vi "Trigger Channel.vi"(8 "error in (no error)":errorcluster, 11 "Node Ptr":T1 format="%.0x") -> (0 "error out":errorcluster)   [LabVIEW 2019, in "Instrument Addon System Explorer.lvlib"]
uses:
  Instrument Addon System Explorer.lvlib
  <vilib>/NI VeriStand/Custom Device API/Custom Device Item Ref.ctl
  NationalInstruments.VeriStand.SystemStorageUI
  Addon Shared/Types/FG Control.ctl
  NationalInstruments.VeriStand.SystemStorage
  Addon Shared/SubVIs/Constants.vi
  <vilib>/NI VeriStand/Custom Device API/NI VeriStand - Get Item Property.vi
  <vilib>/NI VeriStand/Custom Device API/Get Item Property (Boolean).vi
  <vilib>/NI VeriStand/Custom Device API/Get Item Property (String).vi
  <vilib>/NI VeriStand/Custom Device API/NI VeriStand - Set Item Property.vi
  <vilib>/NI VeriStand/Custom Device API/Set Item Property (Boolean).vi
  <vilib>/NI VeriStand/Custom Device API/Set Item Property (String).vi
  <vilib>/NI VeriStand/Custom Device API/Custom Device API.lvlib
  <vilib>/NI VeriStand/UI Controls/Single Node Browser/NI_VS UI Single Node Browser.lvlib
  Addon Shared/Instrument Addon Shared.lvlib
panel:
  in  "Header 2":cluster{"Section Name":string}={"Section Name"="Trigger Item Settings"}
  in  "Channel":refnum<k24>(container) caption="Value"
  in  "Use Channel?":bool
  in  "SHDocVw.IWebBrowser":refnum<k7>(container)
  in  "Header":cluster{"Section Name":string}={"Section Name"="Custom Device Item Settings"}
  in  "Description":string
  out "Name":string
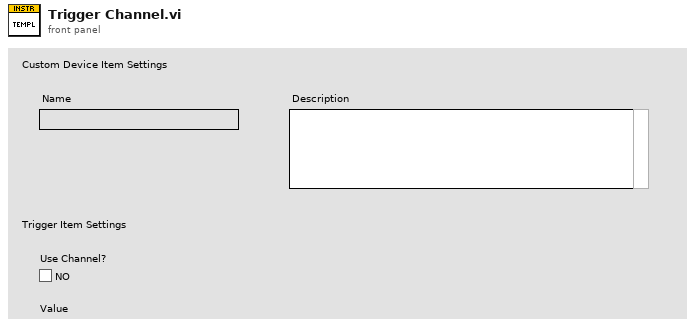
[diagram p1: front panel]
types:
  T1 = typedef "Custom Device API.lvlib/Custom Device Item Ref.ctl" = u64
  T2 = typedef "Instrument Addon Shared.lvlib/FG Control.ctl" = enum16{"Get", "Set"}
  T3 = typedef "Instrument Addon Shared.lvlib/Trigger Parameters.ctl" = cluster{"Use Channel":bool, "Channel Path":string}
  T4 = typedef "Custom Device API.lvlib/Custom Device Item Info.ctl" = cluster{"Name":string, "Is Channel":bool, "GUID":string, "Is Waveform":bool}
  T5 = typedef "Custom Device API.lvlib/Custom Device Commands.ctl" = enum16{"Default", "Item renamed", "Shutdown", "Dynamic button pressed"}
  T6 = typedef "NI_VS UI Single Node Browser.lvlib/Node Ref.ctl" = refnum<k24>
  T7 = typedef "Custom Device API.lvlib/Custom Device Pointer.ctl" = refnum<k24>
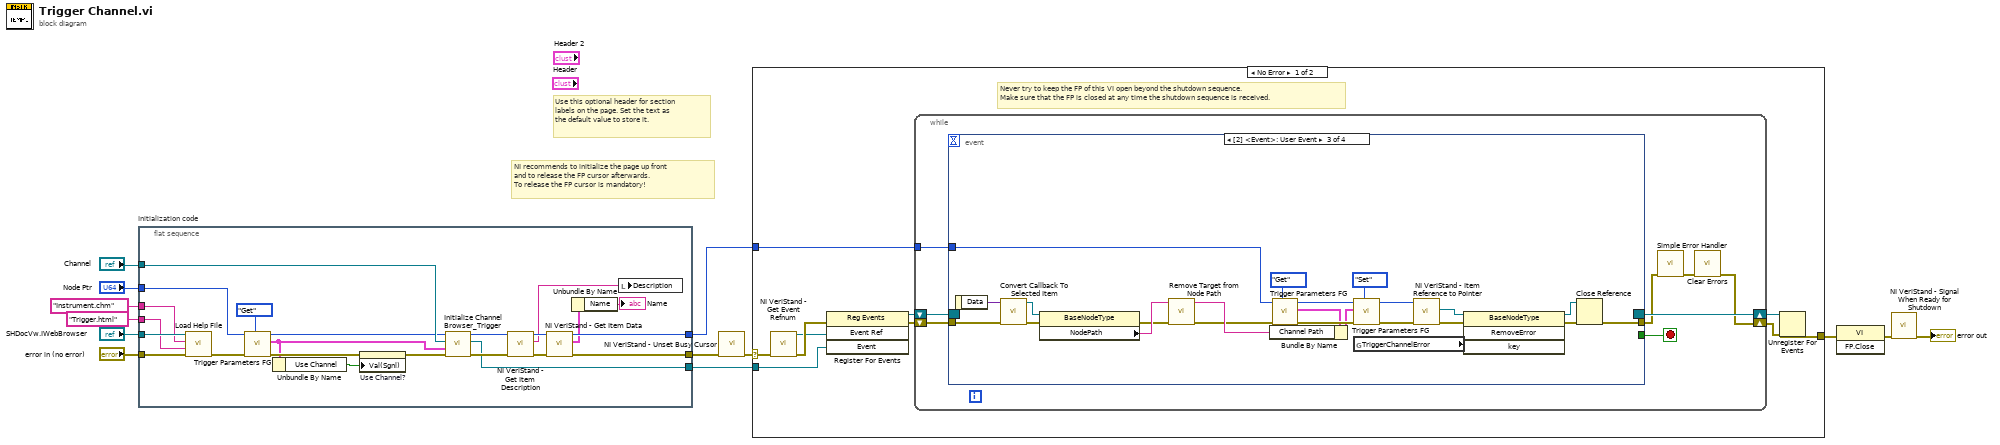
[diagram p0: block diagram]
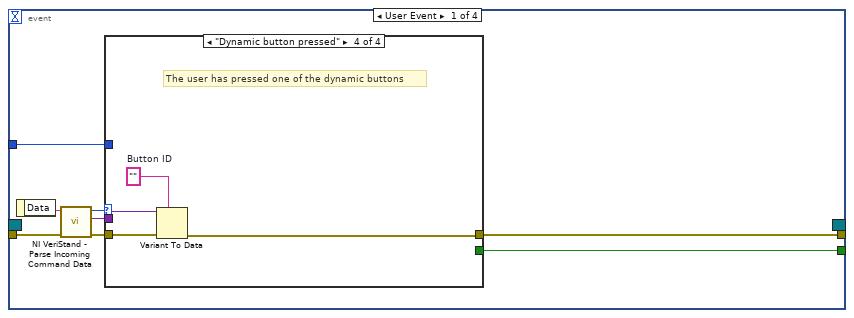
[diagram p2: hidden frame]
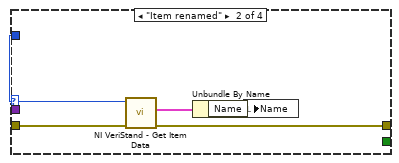
[diagram p4: hidden frame]
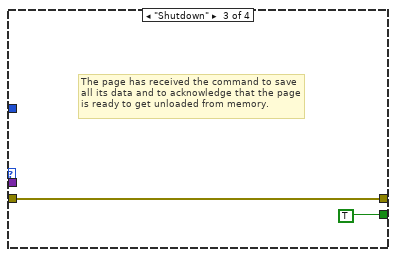
[diagram p5: hidden frame]
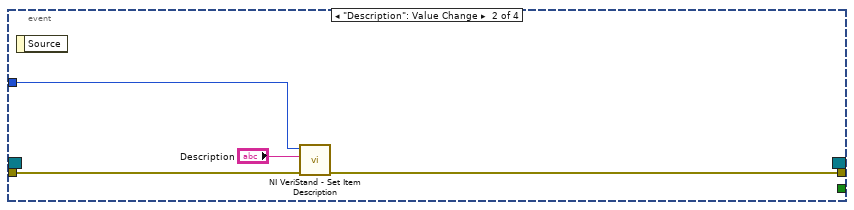
[diagram p6: hidden frame]
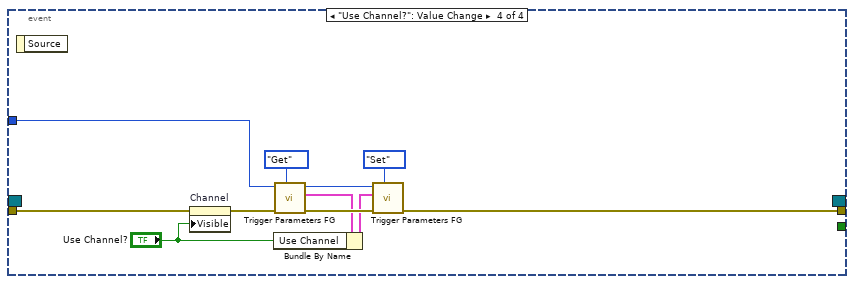
[diagram p7: hidden frame]
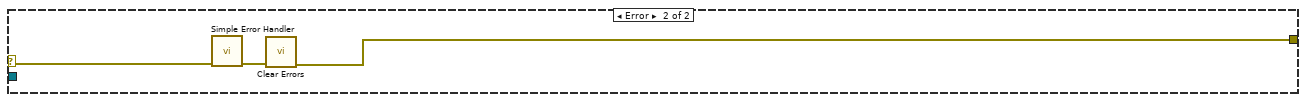
[diagram p8: hidden frame]
diagram:
  # "Use this optional header for section labels on the page. Set the text as the default value to store it."
  # "NI recommends to initialize the page up front\nand to release the FP cursor afterwards.\nTo release the FP cursor is mandatory!"
  n1 = flat-sequence "Initialization code" {
    tunnel: "error in (no error)" -> [w29]
    tunnel: "Node Ptr" -> [w19]
    tunnel: [w31] -> w9
    tunnel: [w36] -> w6
    tunnel: "SHDocVw.IWebBrowser" -> [w28]
    tunnel: "Trigger.html" ("HTML File") -> [w27]
    tunnel: "Instrument.chm" ("Main CHM File") -> [w26]
    tunnel: "Channel" -> [w23]
    tunnel: [w22] -> w1
    frame #0 {
      n2 = call "Load Help File.vi"("error in (no error)"=w29, "HTML File"=w27, "Main CHM File"=w26, "SHDocVw.IWebBrowser2"=w28) -> ("error out"=w20:errorcluster)  [unwired: 7 in]
      n3 = call "Trigger Parameters FG.vi"("Action"=FG_Control."Get", "error in (no error)"=w20, "Item Ref in"=w19) -> ("error out"=w17:errorcluster, "Trigger Parameters"=w14:T3, "Item Ref out"=w18:T1)  [unwired: 6 in]
      n4 = Unbundle By Name(w14) -> ("Use Channel"=w15:bool)
      n5 = property on="Use Channel?" class="Bool (strict)"(error in=w17, "Val(Sgnl)"=w15) -> (error out=w16:errorcluster)  [unwired: 1 in, 1 out]
      n6 = call "Initialize Channel Browser_Trigger.vi"("error in (no error)"=w16, "Trigger Parameters"=w14, ".NET Refnum in"=w23, "Item Ref in"=w18) -> ("error out"=w25:errorcluster, "Event"=w22:refnum<user-event>, "Item Ref out"=w24:T1)  [unwired: 5 in]
      n7 = call <vilib>:"NI VeriStand - Get Item Description.vi"("error in (no error)"=w25, "Item Ref in"=w24) -> ("error out"=w33:errorcluster, "Description"=w34:string, "Item Ref out"=w35:T1)  [unwired: 7 out]
      n8 = call <vilib>:"NI VeriStand - Get Item Data.vi"("error in (no error)"=w33, "Item Ref in"=w35) -> ("error out"=w31:errorcluster, "Item Info"=w32:T4, "Item Ref out"=w36:T1)  [unwired: 7 out]
      n9 = Unbundle By Name(w32) -> ("Name"=→"Name":string)
      n10 = local write "Description"(w34) -> ()
    }
  }
  n11 = call <vilib>:"NI VeriStand - Unset Busy Cursor.vi"("error in (no error)"=w9) -> ("error out"=w8:errorcluster)  [unwired: 10 out]
  n12 = case shown="No Error" w8 {
    selector: w8 -> [w38 w115]
    tunnel: [w43 w113] -> w13
    tunnel: w6 -> [w39 _]
    tunnel: w1 -> [w37 _]
    frame No Error {
      # "Never try to keep the FP of this VI open beyond the shutdown sequence.\nMake sure that the FP is closed at any time the shutdown sequence is received."
      n13 = call <vilib>:"NI VeriStand - Get Event Refnum.vi"("error in (no error)"=w38) -> ("error out"=w46:errorcluster, "Event Ref"=w42:refnum<user-event>)  [unwired: 9 out]
      n14 = register-events(error in=w46, w42, w37) -> (reference out=w40:refnum<event-registration>, error out=w41:errorcluster)  [unwired: 1 in]
      n15 = while {
        tunnel: w39 -> [w50]
        shift-right: [w47] -> w44
        shift-left: w41 -> [w53]
        shift-right: [w54] -> w45
        shift-left: w40 -> [w52]
        stop <- w51 stop-if-true
        n16 = event shown="[2] <Event>: User Event" {
          selector: w52 -> [_ _ _ _]
          dyn-events: [_ _ _ _] -> w54
          timeout: _ -> [_ _ _ _]
          tunnel: w53 -> [w62 w77 w82 w107]
          tunnel: [w58 _ _ _] -> w51
          tunnel: [w57 w76 w83 w102] -> w49
          tunnel: w50 -> [w56 w78 w80 w103]
          event User Event {
            n17 = event-data() -> ("Data"=w61:string)  [unwired: 1 out]
            n18 = call <vilib>:"NI VeriStand - Parse Incoming Command Data.vi"("error in (no error)"=w62, "Incoming data"=w61) -> ("error out"=w60:errorcluster, "Outgoing data"=w55:variant, "Action"=w59:T5)  [unwired: 7 out]
            n19 = case shown="\"Dynamic button pressed\"" w59 {
              tunnel: w60 -> [w63 w68 w69 w74]
              tunnel: [_ _ TRUE _] -> w58
              tunnel: [w63 w65 w69 w71] -> w57
              tunnel: w56 -> [_ w67 _ _]
              tunnel: w55 -> [_ _ _ w73]
              frame "Default", Default {
              }
              frame "Item renamed" {
                n20 = call <vilib>:"NI VeriStand - Get Item Data.vi"("error in (no error)"=w68, "Item Ref in"=w67) -> ("error out"=w65:errorcluster, "Item Info"=w66:T4)  [unwired: 8 out]
                n21 = Unbundle By Name(w66) -> ("Name"=w64:string)
                n22 = local write "Name"(w64) -> ()
              }
              frame "Shutdown" {
                # "The page has received the command to save all its data and to acknowledge that the page is ready to get unloaded from memory."
              }
              frame "Dynamic button pressed" {
                w72 = ""  # Button ID
                # "The user has pressed one of the dynamic buttons"
                n23 = Variant To Data(error in=w74, type=w72, Variant=w73) -> (error out=w71:errorcluster)  [unwired: 1 out]
              }
            }
          }
          event "Description": Value Change {
            n24 = event-data() -> ()  [unwired: 2 out]
            n25 = call <vilib>:"NI VeriStand - Set Item Description.vi"("error in (no error)"=w77, "Description"="Description", "Item Ref in"=w78) -> ("error out"=w76:errorcluster)  [unwired: 8 out]
          }
          event User Event {
            n26 = event-data() -> ("Data"=w81:variant)  [unwired: 1 out]
            n27 = call <vilib>:"Convert Callback To Selected Item.vi"("error in"=w82, "Data"=w81) -> ("error out"=w85:errorcluster, "Selected Item"=w84:T6)  [unwired: 8 in]
            n28 = property class="BaseNodeType"(reference=w84, error in=w85) -> (error out=w91:errorcluster, "NodePath"=w92:string)  [unwired: 1 out]
            n29 = call "Remove Target from Node Path.vi"("error in (no error)"=w91, "NodePath"=w92) -> ("error out"=w93:errorcluster, "PathArrayToString"=w94:string)  [unwired: 8 in]
            n30 = call "Trigger Parameters FG.vi"("Action"=FG_Control."Get", "error in (no error)"=w93, "Item Ref in"=w80) -> ("error out"=w90:errorcluster, "Trigger Parameters"=w88:T3, "Item Ref out"=w89:T1)  [unwired: 6 in]
            n31 = Bundle By Name(cluster=w88, "Channel Path"=w94) -> (w79:T3)
            n32 = call "Trigger Parameters FG.vi"("Action"=FG_Control."Set", "error in (no error)"=w90, "Trigger Parameters"=w79, "Item Ref in"=w89) -> ("error out"=w99:errorcluster, "Item Ref out"=w100:T1)  [unwired: 5 in, 1 out]
            n33 = global read "Constants.vi" "TriggerChannelError"() -> (w101:string)
            n34 = call <vilib>:"NI VeriStand - Item Reference to Pointer.vi"("error in (no error)"=w99, "Item Ref in"=w100) -> ("error out"=w97:errorcluster, "Node Pointer"=w98:T7)  [unwired: 6 in, 2 out]
            n35 = invoke class="BaseNodeType" method="RemoveError"(reference=w98, error in=w97, "key"=w101) -> (reference out=w95:T7, error out=w96:errorcluster)  [unwired: 1 in, 2 out]
            n36 = Close Reference(reference=w95, error in (no error)=w96) -> (error out=w83:errorcluster)
          }
          event "Use Channel?": Value Change {
            n37 = event-data() -> ()  [unwired: 2 out]
            n38 = property on="Channel" class="AXCont"(error in=w107, "Visible"="Use Channel?") -> (error out=w106:errorcluster)  [unwired: 1 in, 1 out]
            n39 = call "Trigger Parameters FG.vi"("Action"=FG_Control."Get", "error in (no error)"=w106, "Item Ref in"=w103) -> ("error out"=w112:errorcluster, "Trigger Parameters"=w110:T3, "Item Ref out"=w111:T1)  [unwired: 6 in]
            n40 = Bundle By Name(cluster=w110, "Use Channel"="Use Channel?") -> (w108:T3)
            n41 = call "Trigger Parameters FG.vi"("Action"=FG_Control."Set", "error in (no error)"=w112, "Trigger Parameters"=w108, "Item Ref in"=w111) -> ("error out"=w102:errorcluster)  [unwired: 5 in, 2 out]
          }
        }
        n42 = call <vilib>:"Simple Error Handler.vi"("error in (no error)"=w49) -> ("error out"=w48:errorcluster)  [unwired: 1 in, 7 out]
        n43 = call <vilib>:"Clear Errors.vi"("error in (no error)"=w48) -> ("error out"=w47:errorcluster)  [unwired: 1 in, 5 out]
      }
      n44 = Unregister For Events(event registration refnum=w45, error in=w44) -> (error out=w43:errorcluster)
    }
    frame Error {
      n45 = call <vilib>:"Simple Error Handler.vi"("error in (no error)"=w115) -> ("error out"=w114:errorcluster)  [unwired: 1 in, 7 out]
      n46 = call <vilib>:"Clear Errors.vi"("error in (no error)"=w114) -> ("error out"=w113:errorcluster)  [unwired: 1 in, 5 out]
    }
  }
  n47 = invoke class="VI" method="FP.Close"(error in=w13) -> (error out=w12:errorcluster)  [unwired: 2 in, 2 out]
  n48 = call <vilib>:"NI VeriStand - Signal When Ready for Shutdown.vi"("error in (no error)"=w12) -> ("error out"=→"error out":errorcluster)  [unwired: 10 out]
